vi "1D Interpolated Table Lookup Booleen.vi"(8 "Min Range":dbl format="%#_13g", 9 "Max Range":dbl=100.0 format="%#_13g", 10 "1d Input Table":bool[](array[boolean]), 11 "Input":dbl=20.0 format="%#_13g") -> (3 "Shift?":bool)   [LabVIEW 2013]
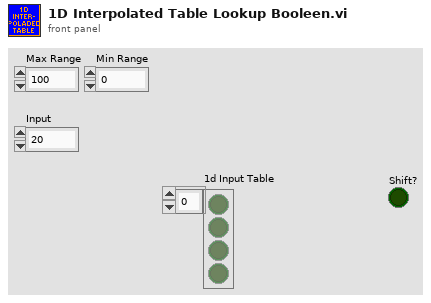
[diagram p1: front panel]
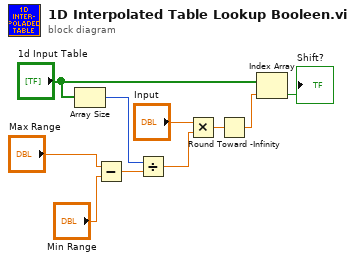
[diagram p0: block diagram]
diagram:
  n1 = Array Size(array="1d Input Table") -> (size(s)=w2:i32)
  n2 = Subtract(x="Max Range", y="Min Range") -> (x-y=w3:dbl)
  n3 = Divide(x=w2, y=w3) -> (x/y=w6:dbl)
  n4 = Multiply(x="Input", y=w6) -> (x*y=w5:dbl)
  n5 = Round Toward -Infinity(1:w5) -> (0:w4:dbl)
  n6 = Index Array(array="1d Input Table", index=w4) -> (element=→"Shift?":bool)
